vi "Pasco Auton Drive.vi"(0 "Desired Heading":dbl, 1 "Measured Heading":dbl, 2 "Time/Distance":dbl, 3 "Power":dbl, 4 "Array Index":i32, 5 "Encoder Distance":dbl, 6 "Increase Power To Each Side":dbl, 7 "Returned Encoder Distance":dbl, 8 "Alloted Off Amount":dbl) -> (14 "Left Drive":dbl, 15 "Right Drive":dbl, 16 "Array Index":i32, 17 "Encoder Out":dbl)   [LabVIEW 2011]
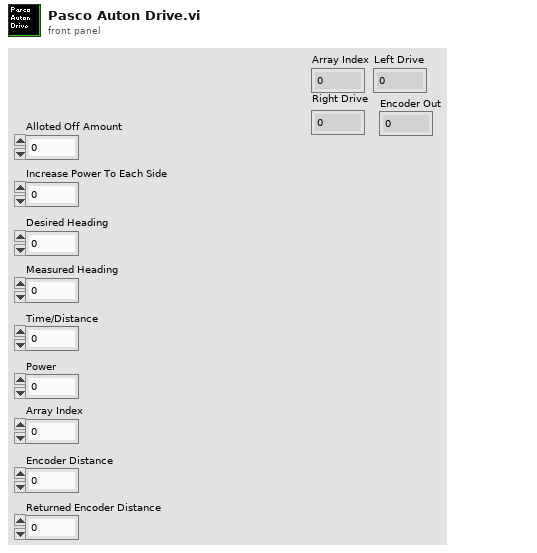
[diagram p1: front panel]
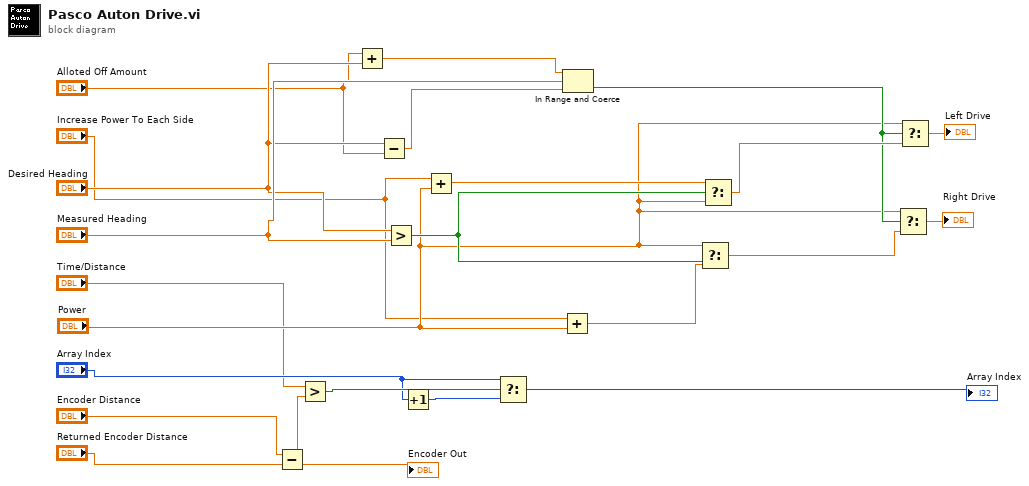
[diagram p0: block diagram]
diagram:
  n1 = Subtract(x="Encoder Distance", y="Returned Encoder Distance") -> (x-y=w12:dbl)
  n2 = Greater?(x="Time/Distance", y=w12) -> (0:w15:bool)
  n3 = Add(x="Alloted Off Amount", y="Desired Heading") -> (x+y=w19:dbl)
  n4 = Subtract(x="Desired Heading", y="Alloted Off Amount") -> (x-y=w20:dbl)
  n5 = Greater?(x="Desired Heading", y="Measured Heading") -> (0:w22:bool)
  n6 = Increment(x="Array Index") -> (x+1=w13:i32)
  n7 = Add(x="Increase Power To Each Side", y="Power") -> (x+y=w23:dbl)
  n8 = Select(t="Array Index", s=w15, f=w13) -> (s? t:f=→"Array Index":i32)
  n9 = Add(x="Increase Power To Each Side", y="Power") -> (x+y=w21:dbl)
  n10 = In Range and Coerce(upper limit=w19, x="Measured Heading", lower limit=w20) -> (In Range?=w17:bool)  [unwired: 1 out]
  n11 = Select(t="Power", s=w22, f=w21) -> (s? t:f=w16:dbl)
  n12 = Select(t=w23, s=w22, f="Power") -> (s? t:f=w18:dbl)
  n13 = Select(t="Power", s=w17, f=w16) -> (s? t:f=→"Right Drive":dbl)
  n14 = Select(t="Power", s=w17, f=w18) -> (s? t:f=→"Left Drive":dbl)
  "Encoder Out" <- "Returned Encoder Distance"
